vi "Filtr_sumu_pro_okno.vi"(0 "trig_in":bool=TRUE, 1 "i":i32, 2 "Citlivost 2":i32, 3 "BShitftIn":i32, 4 "ShiftIn":bool) -> (5 "trig_out":bool=TRUE, 6 "ShiftOut":bool, 7 "BShiftOut":i32)   [LabVIEW 2019]
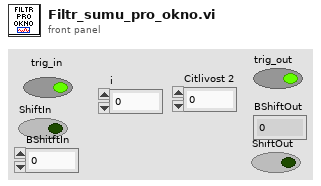
[diagram p1: front panel]
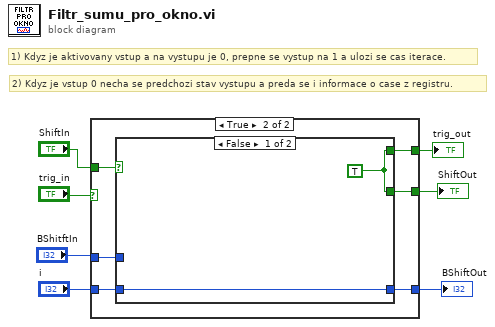
[diagram p0: block diagram]
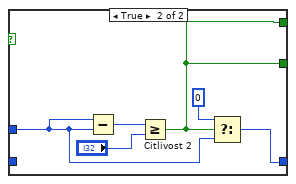
[diagram p3: hidden frame]
diagram:
  # "2) Kdyz je vstup 0 necha se predchozi stav vystupu a preda se i informace o case z registru."
  # "1) Kdyz je aktivovany vstup a na vystupu je 0, prepne se vystup na 1 a ulozi se cas iterace."
  n1 = case shown="True" "trig_in" {
    tunnel: [w9 w15] -> w6
    tunnel: "i" -> [_ w14]
    tunnel: [w8 w13] -> w2
    tunnel: [w9 w12] -> w4
    tunnel: "ShiftIn" -> [w9 w11]
    tunnel: "BShitftIn" -> [w8 w10]
    frame False {
    }
    frame True {
      n2 = case shown="False" w11 {
        tunnel: [w16 w21] -> w15
        tunnel: w14 -> [w17 _]
        tunnel: [w17 w20] -> w13
        tunnel: [w16 w21] -> w12
        tunnel: w10 -> [_ w18]
        frame False {
          w16 = TRUE
        }
        frame True {
          n3 = Subtract(x=w18, y=w18) -> (x-y=w23:i32)
          n4 = Greater Or Equal?(x=w23, y="Citlivost 2") -> (x >= y?=w21:bool)
          n5 = Select(t=0, s=w21, f=w18) -> (s? t:f=w20:i32)
        }
      }
    }
  }
  "trig_out" <- w6
  "ShiftOut" <- w4
  "BShiftOut" <- w2
